vi "Tare.vi"(8 "error in (no error)":errorcluster caption="entrée d'erreur (pas d'erreur)", 11 "Class Balance_Adam_GBK en entrée":refnum<class "Class Balance_Adam_GBK.lvclass">) -> (0 "error out":errorcluster caption="sortie d'erreur", 3 "Class Balance_Adam_GBK en sortie":refnum<class "Class Balance_Adam_GBK.lvclass">)   [LabVIEW 2020, in "Library Instrument & Equipement.lvlib" / "Library Balance.lvlib" / "Class Balance_Adam_GBK.lvclass"]
uses:
  Class Balance_Adam_GBK.lvclass
  Class Balance_Adam_GBK.lvclass/Class Balance_Adam_GBK.ctl
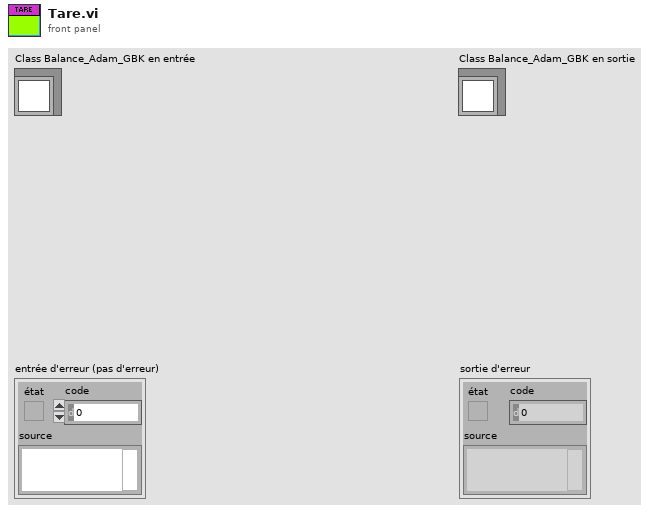
[diagram p1: front panel]
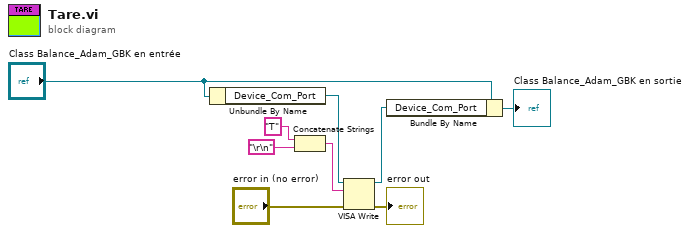
[diagram p0: block diagram]
diagram:
  n1 = Unbundle By Name("Class Balance_Adam_GBK en entrée") -> ("Device_Com_Port"=w9:refnum<visa-resource-name>)
  n2 = Concatenate Strings("T" ("chaîne"), "\r\n") -> (w6:string)
  n3 = VISA Write(VISA resource name=w9, write buffer=w6, error in (no error)="error in (no error)") -> (VISA resource name out=w3:refnum<visa-resource-name>, error out=→"error out":errorcluster)  [unwired: 1 out]
  n4 = Bundle By Name(cluster="Class Balance_Adam_GBK en entrée", "Device_Com_Port"=w3) -> (→"Class Balance_Adam_GBK en sortie":refnum<class "Class Balance_Adam_GBK.lvclass">)
